vi "Select_Filename_List.vi"(4 "No dialogs":bool, 5 "File Type":string, 6 "Search String":string, 7 "At Dialog Prompt Post Process":T1, 8 "Previous Choice":path) -> (0 "Current Results filenames":path[](array[path]), 1 "Selected files":path[](array[path]), 3 "Choosen path":path)   [LabVIEW 2016]
uses:
  Controls/File_Selector_Type.ctl
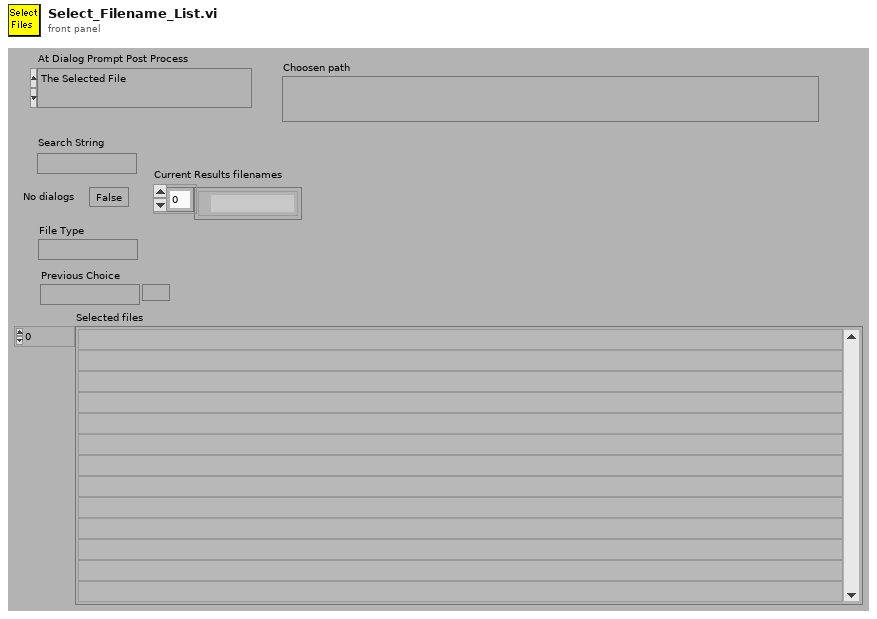
[diagram p1: front panel]
types:
  T1 = typedef "File_Selector_Type.ctl" = enum16{"The Selected File", "The Selected Folder", "Files containing the search string in the selected folder", "All files listed in selected file"}
  T2 = enum32{"existing file", "new file", "new or existing file", "existing dir", "new dir", "new or existing dir", "existing file (use LLBs)", "new file (use LLBs)", "new or existing file (use LLBs)", "new or existing file or directory (use LLBs)"}
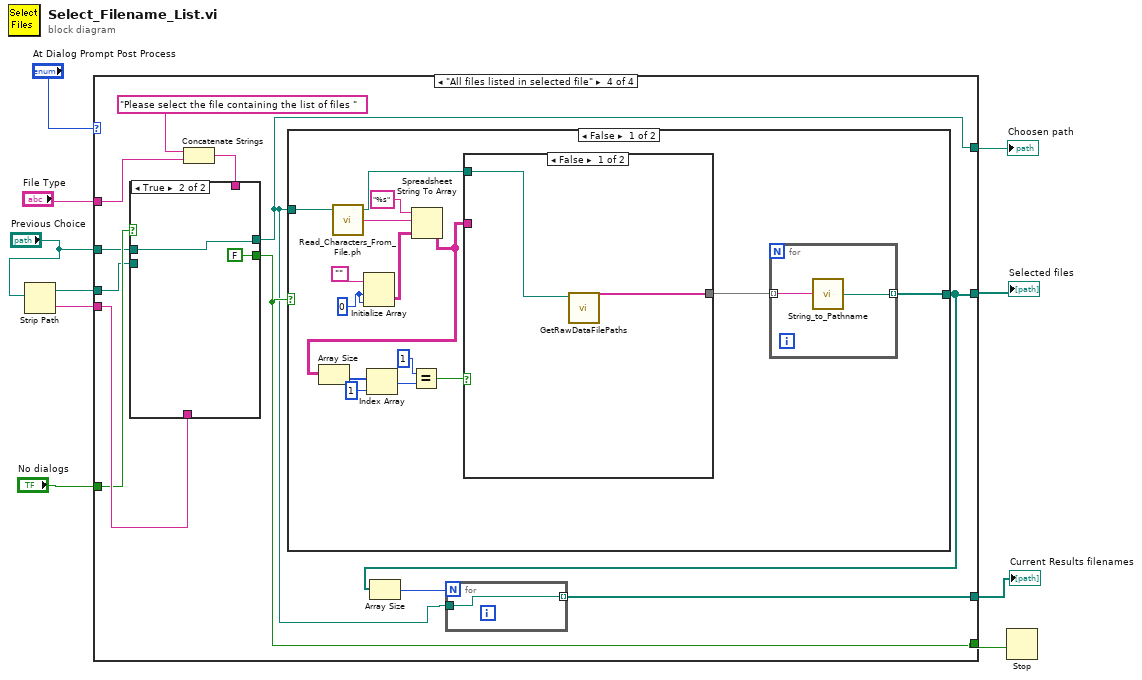
[diagram p0: block diagram]
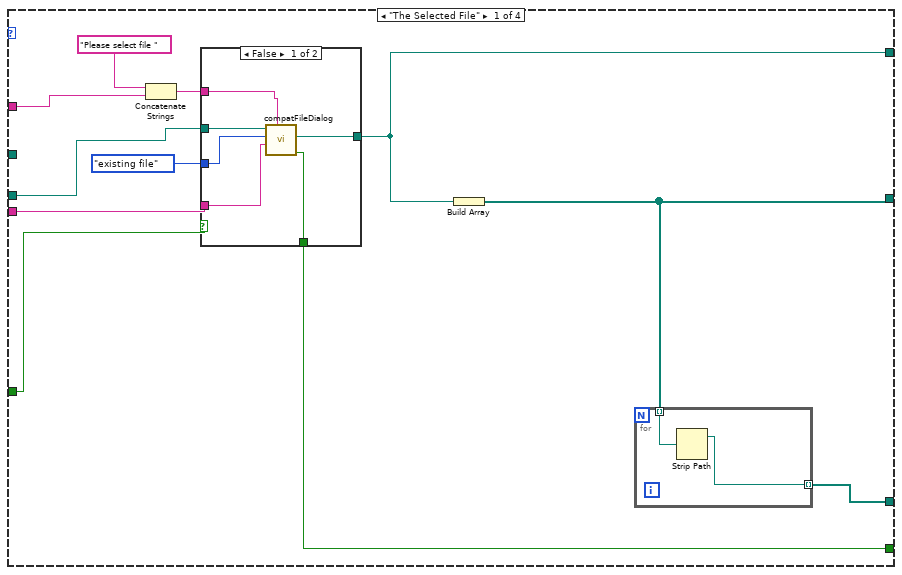
[diagram p2: hidden frame]
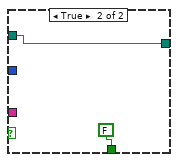
[diagram p3: hidden frame]
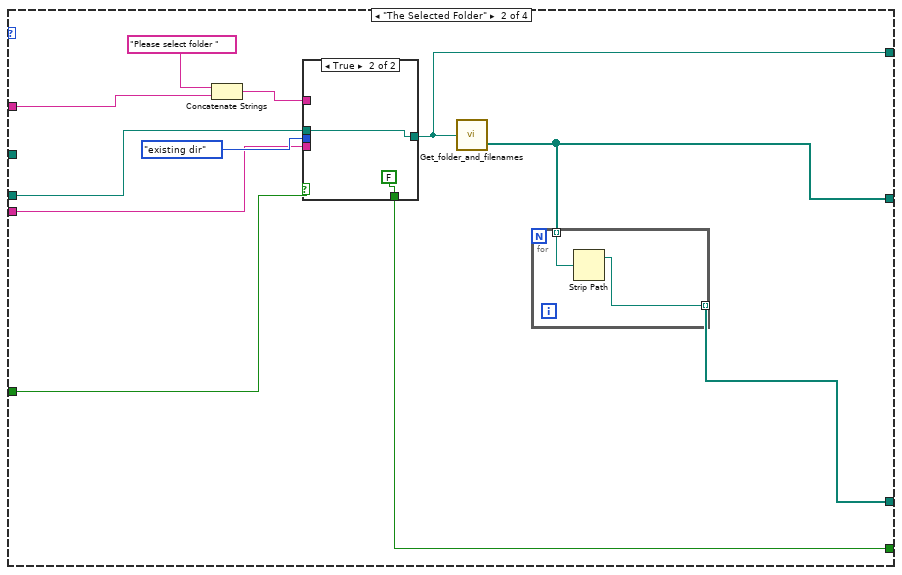
[diagram p4: hidden frame]
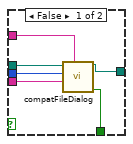
[diagram p5: hidden frame]
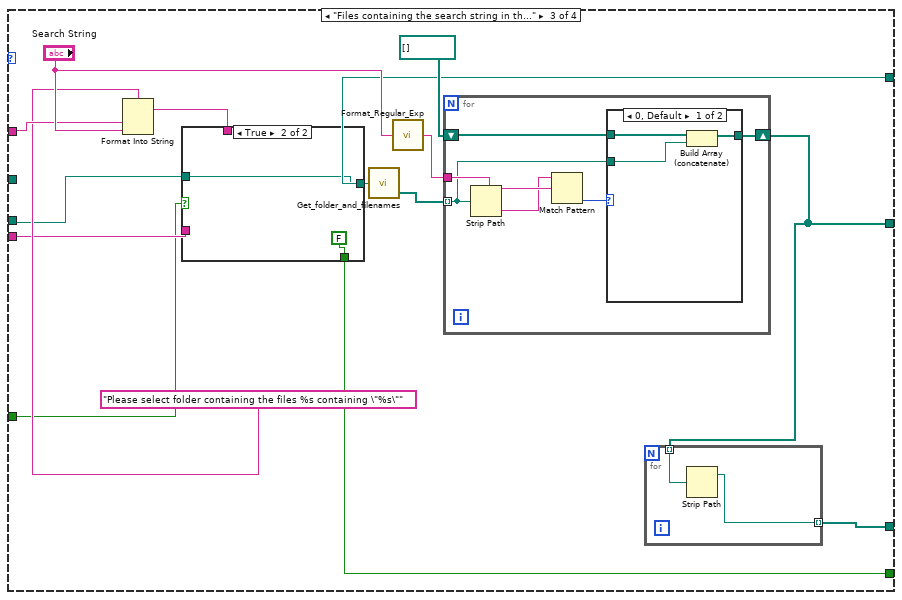
[diagram p6: hidden frame]
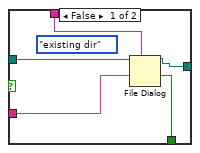
[diagram p7: hidden frame]
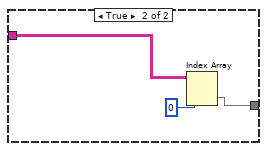
[diagram p9: hidden frame]
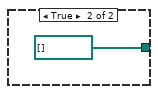
[diagram p10: hidden frame]
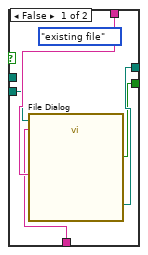
[diagram p11: hidden frame]
diagram:
  n1 = Strip Path(path="Previous Choice") -> (stripped path=w6:path, name=w5:string)
  n2 = case shown="\"All files listed in selected file\"" "At Dialog Prompt Post Process" {
    tunnel: [w12 w33 w53 w90] -> w7
    tunnel: "File Type" -> [w20 w40 w60 w96]
    tunnel: [w17 w41 w61 w91] -> w8
    tunnel: w6 -> [w16 w37 w58 w92]
    tunnel: w5 -> [w15 w36 w57 w94]
    tunnel: [w13 w35 w56 w87] -> w4
    tunnel: "No dialogs" -> [w14 w34 w55 w93]
    tunnel: [w11 w32 w54 w88] -> w2
    tunnel: "Previous Choice" -> [_ _ _ w86]
    frame "The Selected File" {
      n3 = Concatenate Strings("Please select file " ("prompt"), w20) -> (w18:string)
      n4 = case shown="False" w14 {
        tunnel: T2."existing file" ("select mode (2)") -> [w29 _]
        tunnel: w18 -> [w28 _]
        tunnel: [w27 FALSE ("cancelled")] -> w17
        tunnel: w16 -> [w26 w31]
        tunnel: w15 -> [w25 _]
        tunnel: [w24 w31] -> w13
        frame False {
          n5 = call <vilib>:"compatFileDialog.vi"("prompt"=w28, "default name"=w25, "select mode (2)"=w29, "start path"=w26) -> ("cancelled"=w27:bool, "path"=w24:path)  [unwired: 3 in, 3 out]
        }
        frame True {
        }
      }
      n6 = Build Array(w13) -> (w12:path[])
      n7 = for {
        tunnel: w12 -> [w23] mode=indexing
        tunnel: [w22] -> w11 mode=indexing
        n8 = Strip Path(path=w23) -> (stripped path=w22:path)  [unwired: 1 out]
      }
    }
    frame "The Selected Folder" {
      n9 = Concatenate Strings("Please select folder " ("prompt"), w40) -> (w38:string)
      n10 = case shown="True" w34 {
        tunnel: T2."existing dir" ("select mode (2)") -> [w50 _]
        tunnel: [w49 FALSE ("cancelled")] -> w41
        tunnel: w38 -> [w48 _]
        tunnel: w37 -> [w47 w52]
        tunnel: w36 -> [w46 _]
        tunnel: [w45 w52] -> w35
        frame False {
          n11 = call <vilib>:"compatFileDialog.vi"("prompt"=w48, "default name"=w46, "select mode (2)"=w50, "start path"=w47) -> ("cancelled"=w49:bool, "path"=w45:path)  [unwired: 3 in, 3 out]
        }
        frame True {
        }
      }
      n12 = call "Get_folder_and_filenames.vi"("file path (dialog if empty)"=w35) -> ("Files"=w33:path[])  [unwired: 1 out]
      n13 = for {
        tunnel: w33 -> [w44] mode=indexing
        tunnel: [w43] -> w32 mode=indexing
        n14 = Strip Path(path=w44) -> (stripped path=w43:path)  [unwired: 1 out]
      }
    }
    frame "Files containing the search string in the selected folder" {
      n15 = Format Into String(format string="Please select folder containing the files %s containing \"%s\"" ("prompt"), w60, "Search String") -> (resulting string=w66:string)  [unwired: 2 in, 1 out]
      n16 = case shown="True" w55 {
        tunnel: w66 -> [w73 _]
        tunnel: [w72 FALSE ("cancelled")] -> w61
        tunnel: w58 -> [w71 w75]
        tunnel: w57 -> [w70 _]
        tunnel: [w69 w75] -> w56
        frame False {
          (unwired) T2."existing dir" ("select mode (2)")
          n17 = File Dialog(7:w73, 9:w70, 11:w71) -> (1:w72:bool, 3:w69:path)  [unwired: 1 in, 5 out]
        }
        frame True {
        }
      }
      n18 = call "Get_folder_and_filenames.vi"("file path (dialog if empty)"=w56) -> ("Files"=w65:path[])  [unwired: 1 out]
      n19 = call "Format_Regular_Exp.vi"("Regular expression"="Search String") -> ("Case Insensitive for html"=w62:string)
      n20 = for {
        shift-right: [w76] -> w53
        shift-left: path[] [] -> [w78]
        tunnel: w62 -> [w81]
        tunnel: w65 -> [w77] mode=indexing
        n21 = Strip Path(path=w77) -> (name=w80:string)  [unwired: 1 out]
        n22 = Match Pattern(string=w80, regular expression=w81) -> (offset past match=w79:i32)  [unwired: 4 out]
        n23 = case shown="0, Default" w79 {
          tunnel: w78 -> [w84 w85]
          tunnel: w77 -> [w83 _]
          tunnel: [w82 w85] -> w76
          frame 0, Default {
            n24 = Build Array (concatenate)(w84, w83) -> (w82:path[])
          }
          frame -1 {
          }
        }
      }
      n25 = for {
        tunnel: w53 -> [w68] mode=indexing
        tunnel: [w67] -> w54 mode=indexing
        n26 = Strip Path(path=w68) -> (stripped path=w67:path)  [unwired: 1 out]
      }
    }
    frame "All files listed in selected file" {
      n27 = Concatenate Strings("Please select the file containing the list of files " ("prompt"), w96) -> (w95:string)
      n28 = case shown="True" w93 {
        tunnel: [w122 FALSE ("cancelled")] -> w91
        tunnel: w95 -> [w126 _]
        tunnel: w92 -> [w124 _]
        tunnel: w94 -> [w125 _]
        tunnel: [w123 w127] -> w87
        tunnel: w86 -> [_ w127]
        frame False {
          (unwired) T2."existing file" ("select mode (2)")
          n29 = call "File Dialog"("start path"=w124, "prompt"=w126, "default name"=w125) -> ("selected path"=w123:path, "cancelled"=w122:bool)  [unwired: 9 in, 2 out]
        }
        frame True {
        }
      }
      n30 = case shown="False" w91 {
        tunnel: w87 -> [w102 _]
        tunnel: [w100 path[] []] -> w90
        frame False {
          w109 = 0 ("Dimension Size")
          n31 = call "Read_Characters_From_File.ph.vi"("file path (dialog if empty)"=w102) -> ("new file path (NotAPath if cancelled)"=w99:path, "character string"=w113:string)  [unwired: 1 in, 6 out]
          n32 = Initialize Array("", w109, w109) -> (w111:string[][])
          n33 = Spreadsheet String To Array(format string="%s", spreadsheet string=w113, array type (2D Dbl)=w111) -> (array=w108:string[][])  [unwired: 1 out]
          n34 = Array Size(array=w108) -> (size(s)=w107:i32[])
          n35 = Index Array(array=w107, index=1) -> (element=w105:i32)
          n36 = Equal?(x=1, y=w105) -> (x = y?=w103:bool)
          n37 = case shown="False" w103 {
            tunnel: w108 -> [_ w120]
            tunnel: w99 -> [w117 _]
            tunnel: [w116 w118] -> w101
            frame False {
              n38 = call "GetRawDataFilePaths.vi"("Results file or Folder"=w117) -> ("RawDataFilePaths"=w116:string[])  [unwired: 9 in, 1 out]
            }
            frame True {
              n39 = Index Array(array=w120, index (col)=0 ("disabled index (col)")) -> (element=w118:string[])  [unwired: 1 in]
            }
          }
          n40 = for {
            tunnel: w101 -> [w115] mode=indexing
            tunnel: [w114] -> w100 mode=indexing
            n41 = call "String_to_Pathname.vi"("Input String"=w115) -> ("path"=w114:path)
          }
        }
        frame True {
        }
      }
      n42 = Array Size(array=w90) -> (size(s)=w89:i32)
      n43 = for {
        N: w89 -> [_]
        tunnel: [w98] -> w88 mode=indexing
        tunnel: w87 -> [w98]
      }
    }
  }
  "Selected files" <- w7
  "Choosen path" <- w4
  "Current Results filenames" <- w2
  n44 = Stop(stop? (T)=w8) -> ()
